vi "CMD_Reset.vi"(1 "Line":string="encoders") -> (0 "Done":bool=TRUE)   [LabVIEW 2017, in "Apple script.lvlib"]
uses:
  Apple script.lvlib
  Support Code/Support Code.lvlib
panel:
  in  "Parameters":i32[](array[numeric])=[0, 0]
  in  "Subcommands":string[](array[string])=["encoders", "gyro"]
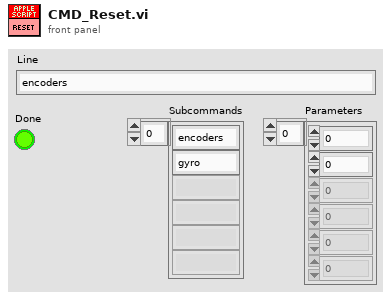
[diagram p1: front panel]
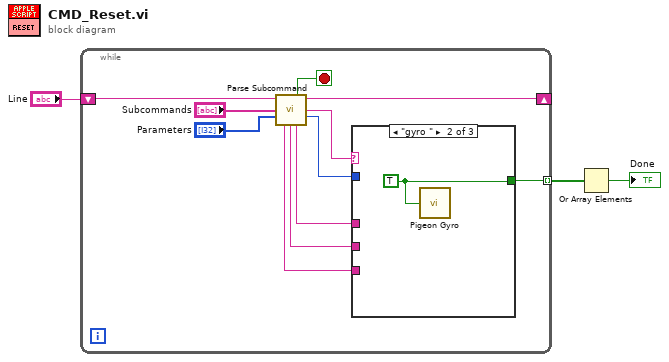
[diagram p0: block diagram]
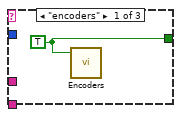
[diagram p2: hidden frame]
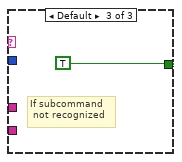
[diagram p3: hidden frame]
diagram:
  n1 = while {
    shift-right: [w11] -> _
    shift-left: "Line" -> [w14]
    tunnel: [w4] -> w2 mode=indexing
    stop <- w10 stop-if-true
    n2 = call "Parse Subcommand.vi"("Text In"=w14, "Subcommands"="Subcommands", "Parameters"="Parameters") -> ("Done"=w10:bool, "Text Out"=w11:string, "Subcommand"=w9:string, "# of Parameters"=w8:i32, "Parameter 3"=w5:string, "Parameter 2"=w6:string, "Parameter 1"=w7:string)  [unwired: 6 in]
    n3 = case shown="\"gyro \"" w9 {
      tunnel: w8 -> [_ _ _]
      tunnel: w7 -> [_ _ _]
      tunnel: w6 -> [_ _ _]
      tunnel: w5 -> [_ _ _]
      tunnel: [w15 w16 TRUE] -> w4
      frame "encoders" {
        w15 = TRUE ("Reset Encoders?")
        n4 = call "Encoders.vi"("Reset Encoders?"=w15) -> ()  [unwired: 2 in, 4 out]
      }
      frame "gyro " {
        w16 = TRUE
        n5 = call "Pigeon Gyro.vi"("Reset Yaw?"=w16) -> ()  [unwired: 2 out]
      }
      frame Default {
        # "If subcommand\n not recognized"
      }
    }
  }
  n6 = Or Array Elements(Boolean array=w2) -> (logical OR=→"Done":bool)
